vi "configure.vi"(8 "error in (no error)":errorcluster, 11 "DL090602SutterMP285Stage in":refnum<class "StageMMS2015ASI.lvclass">) -> (0 "error out":errorcluster, 3 "DL090602SutterMP285Stage out":refnum<class "StageMMS2015ASI.lvclass">)   [LabVIEW 2010, in "StageMMS2015ASI.lvclass"]
doc: "The dynamic dispatch version of this VI loads and displays the configuration file associated with the plug-in object. The user modify and save the configuration data."
uses:
  StageMMS2015ASI.lvclass
  StageMMS2015ASI.lvclass/StageMMS2015ASI.ctl
  common/classes/GenericComponent/GenericComponent/GenericComponent.lvclass
panel:
  in  "Step Factor":dbl[unit]
  in  "Speed":dbl[unit]
  out "Configuration":string
  in  "cancel button":bool
  in  "save button":bool
  in  "Serial port name":refnum<visa-resource-name>
  # "Configure DL090602SutterMP285Stage"
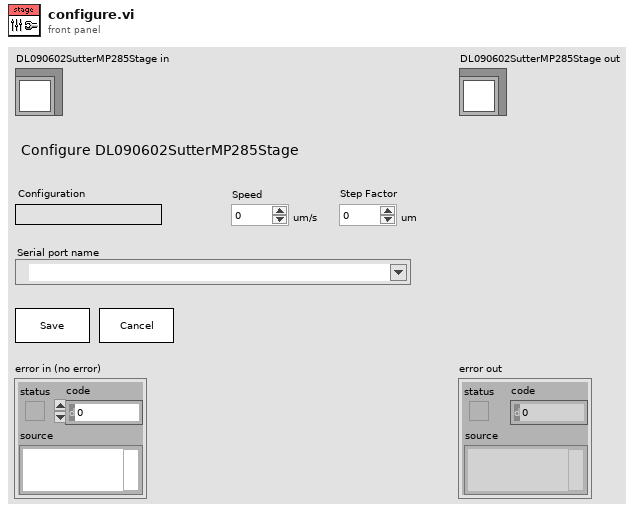
[diagram p1: front panel]
types:
  T1 = typedef "StageMMS2015ASI.lvclass/status_cluster.ctl" = cluster{"STEP_DIV":i32, "STEP_MUL":i32, "XSPEED":i32, "VERSION":i32}
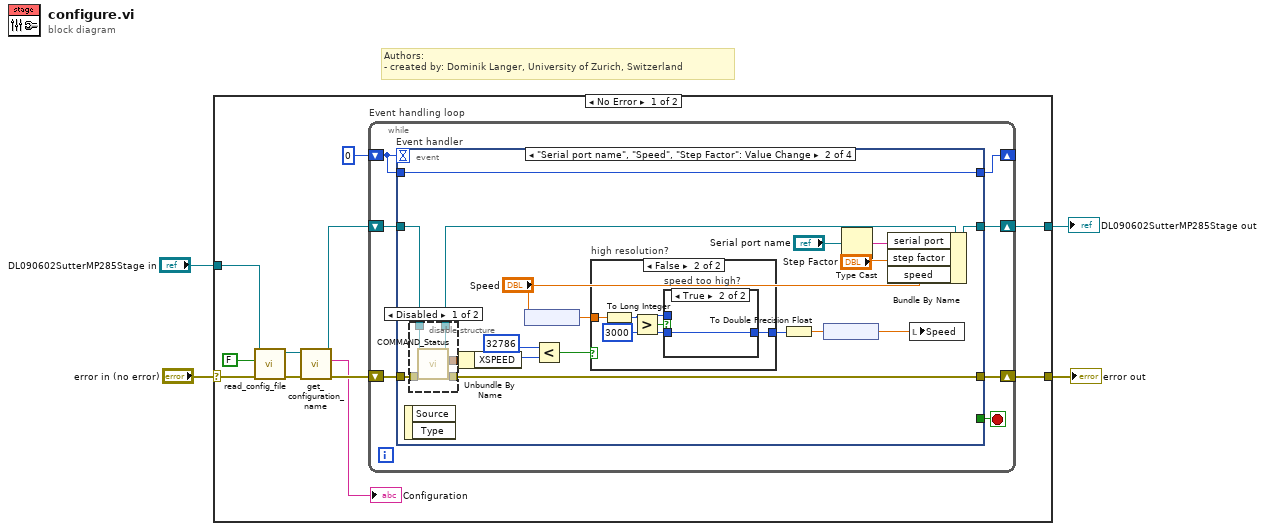
[diagram p0: block diagram]
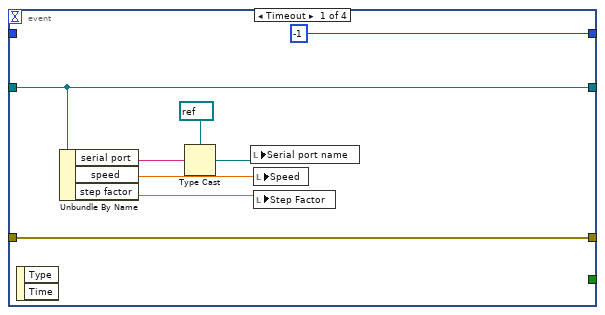
[diagram p2: hidden frame]
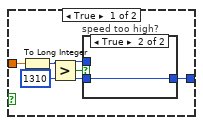
[diagram p4: hidden frame]
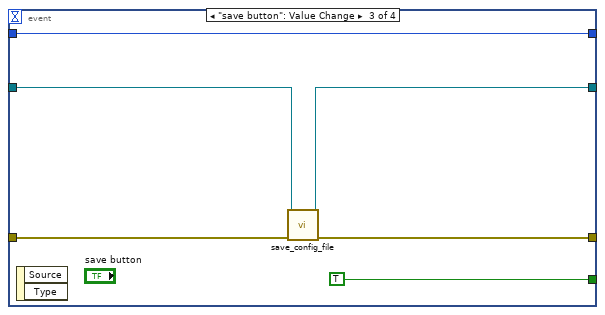
[diagram p7: hidden frame]
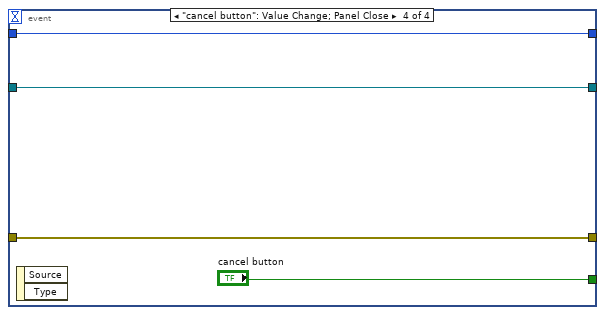
[diagram p8: hidden frame]
diagram:
  # "Authors: \n- created by: Dominik Langer, University of Zurich, Switzerland"
  n1 = case shown="No Error" "error in (no error)" {
    selector: "error in (no error)" -> [w12 w81]
    tunnel: [w15 w81] -> w3
    tunnel: "DL090602SutterMP285Stage in" -> [w11 w80]
    tunnel: [w14 w80] -> w1
    frame No Error {
      n2 = call-dynamic "read_config_file.vi"("error in (no error)"=w12, "force load?"=FALSE, "GenericPlugin in"=w11) -> ("error out"=w9:errorcluster, "GenericPlugin out"=w7:refnum<class "StageMMS2015ASI.lvclass">)  [unwired: 7 out]
      n3 = call "get_configuration_name.vi"("error in (no error)"=w9, "GenericPlugin.lvclass in"=w7) -> ("error out"=w8:errorcluster, "configuration name"=→"Configuration":string, "GenericPlugin.lvclass out"=w6:refnum<class "StageMMS2015ASI.lvclass">)  [unwired: 7 in]
      n4 = while "Event handling loop" {
        shift-right: [w20] -> w15
        shift-left: w8 -> [w22]
        shift-right: [w19] -> w14
        shift-left: w6 -> [w21]
        shift-right: [w17] -> _
        shift-left: 0 -> [w18]
        stop <- w16 stop-if-true
        n5 = event "Event handler" shown="[1] \"Serial port name\", \"Speed\", \"Step Factor\": Value Change" {
          selector: _ -> [_ _ _ _]
          dyn-events: _ -> [_ _ _ _]
          timeout: w18 -> [_ _ _ _]
          tunnel: w22 -> [w30 w44 w73 w79]
          tunnel: w21 -> [w28 w42 w71 w78]
          tunnel: [w30 w36 w72 w79] -> w20
          tunnel: [w28 w46 w70 w78] -> w19
          tunnel: [-1 w48 w75 w77] -> w17
          tunnel: w18 -> [_ w48 w75 w77]
          tunnel: [_ _ TRUE "cancel button"] -> w16
          event Timeout {
            n6 = event-data() -> ()  [unwired: 3 out]
            n7 = Unbundle By Name(w28) -> ("serial port"=w27:string, "speed"=w24:dbl[unit], "step factor"=w23:dbl[unit])
            n8 = Type Cast(type=refnum<visa-resource-name> refnum ("Serial port name"), x=w27) -> (*(type *) &x=w26:refnum<visa-resource-name>)
            n9 = local write "Serial port name"(w26) -> ()
            n10 = local write "Speed"(w24) -> ()
            n11 = local write "Step Factor"(w23) -> ()
          }
          event "Serial port name", "Speed", "Step Factor": Value Change {
            n12 = event-data() -> ()  [unwired: 3 out]
            n13 = disable-structure shown="Disabled" {
              disable-tunnel: w44 -> [w53 w54]
              disable-tunnel: [w52 _] -> w43
              disable-tunnel: w42 -> [w51 w55]
              disable-tunnel: [w50 w55] -> w41
              disable-tunnel: [w49 w54] -> w36
              frame Disabled {
                n14 = call-dynamic "COMMAND_Status.vi"("error in (no error)"=w53, "StageDL090602SutterMP285 in"=w51) -> ("error out"=w49:errorcluster, "status"=w52:T1, "StageDL090602SutterMP285 out"=w50:refnum<class "StageMMS2015ASI.lvclass">)  [unwired: 7 in]
              }
              frame Enabled {
              }
            }
            n15 = Unbundle By Name(w43) -> ("XSPEED"=w39:i32)
            n16 = node("Speed") -> (w37:dbl)
            n17 = Less?(x=32786, y=w39) -> (x < y?=w40:bool)
            n18 = case "high resolution?" shown="False" w40 {
              tunnel: w37 -> [w59 w66]
              tunnel: [w56 w63] -> w34
              frame True {
                w58 = 1310
                n19 = To Long Integer(number=w59) -> (32bit integer=w57:i32)
                n20 = Greater?(x=w57, y=w58) -> (0:w60:bool)
                n21 = case "speed too high?" shown="True" w60 {
                  tunnel: w58 -> [_ w62]
                  tunnel: [w61 w62] -> w56
                  tunnel: w57 -> [w61 _]
                  frame False {
                  }
                  frame True {
                  }
                }
              }
              frame False {
                w65 = 3000
                n22 = To Long Integer(number=w66) -> (32bit integer=w64:i32)
                n23 = Greater?(x=w64, y=w65) -> (0:w67:bool)
                n24 = case "speed too high?" shown="True" w67 {
                  tunnel: w65 -> [_ w69]
                  tunnel: [w68 w69] -> w63
                  tunnel: w64 -> [w68 _]
                  frame False {
                  }
                  frame True {
                  }
                }
              }
            }
            n25 = To Double Precision Float(number=w34) -> (double precision float=w33:dbl)
            n26 = node(w33) -> (w32:dbl[unit])
            n27 = Type Cast(x="Serial port name") -> (*(type *) &x=w45:string)  [unwired: 1 out]
            n28 = Bundle By Name(cluster=w41, "serial port"=w45, "step factor"="Step Factor", "speed"="Speed") -> (w46:refnum<class "StageMMS2015ASI.lvclass">)
            n29 = local write "Speed"(w32) -> ()
          }
          event "save button": Value Change {
            n30 = event-data() -> ()  [unwired: 3 out]
            n31 = call-dynamic "save_config_file.vi"("error in (no error)"=w73, "GenericPlugin in"=w71) -> ("error out"=w72:errorcluster, "GenericPlugin out"=w70:refnum<class "StageMMS2015ASI.lvclass">)  [unwired: 1 in, 7 out]
          }
          event "cancel button": Value Change; Panel Close {
            n32 = event-data() -> ()  [unwired: 3 out]
          }
        }
      }
    }
    frame Error {
    }
  }
  "error out" <- w3
  "DL090602SutterMP285Stage out" <- w1
